vi "PC_of_IP.vi"(8 "error in (no error)":errorcluster, 10 "EndPoint":string) -> (0 "error out":errorcluster, 2 "IP/Endpoint":string)   [LabVIEW 2016]
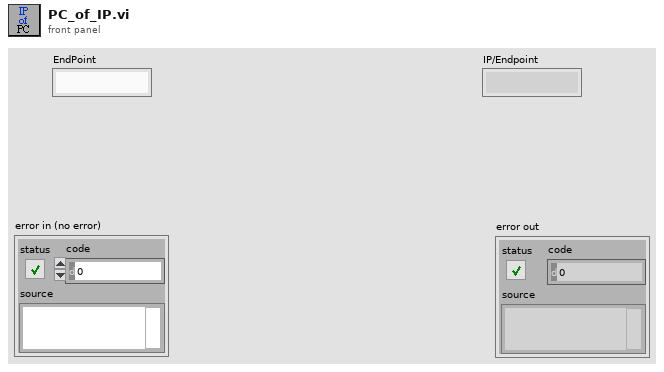
[diagram p1: front panel]
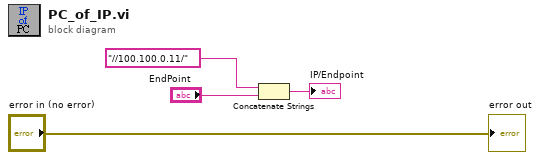
[diagram p0: block diagram]
diagram:
  n1 = Concatenate Strings("//100.100.0.11/", "EndPoint") -> (→"IP/Endpoint":string)
  "error out" <- "error in (no error)"
